vi "Create Counter PWM Input Module.vi"   [LabVIEW 2017, in "Scan Engine Scripting.lvlib"]
uses:
  Scan Engine Scripting.lvlib
  NI 9423/NI 9423.lvclass
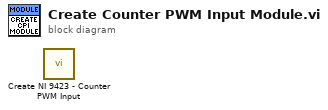
[diagram p0: block diagram]
diagram:
  n1 = call "Create NI 9423 - Counter PWM Input.vi"() -> ()  [unwired: 10 in, 2 out]
